vi "BallSub.vi"(6 "Ball Ref":cluster{refnum<vi>, "PaneColor":u32}[](array[cluster]), 8 "Cluster width":i32=200, 9 "Ball Nr":i32, 10 "Ball Refs":refnum<vi>[](array[refnum]), 11 "Position In":i32) -> (3 "Position out":i32)   [LabVIEW 2014]
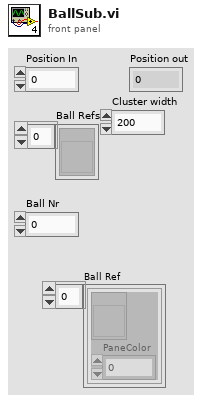
[diagram p1: front panel]
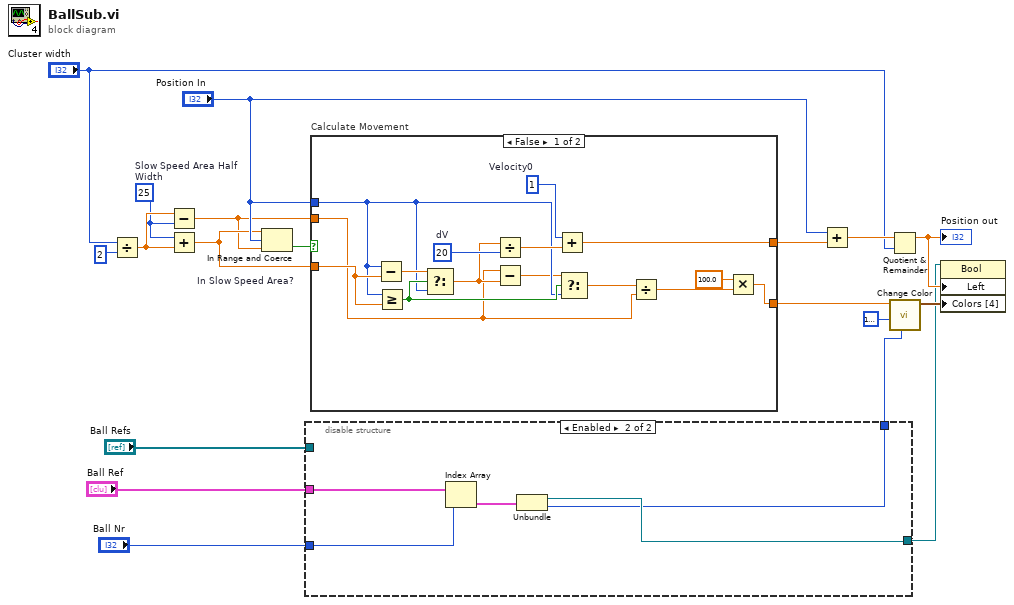
[diagram p0: block diagram]
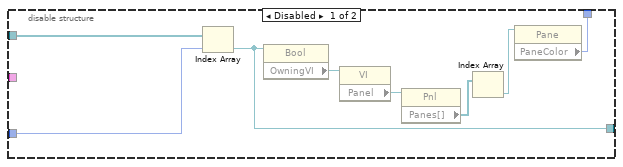
[diagram p2: hidden frame]
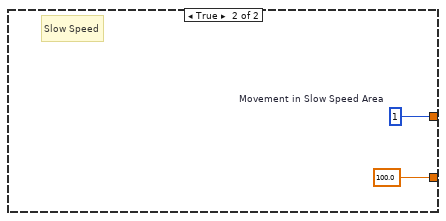
[diagram p3: hidden frame]
diagram:
  w8 = 25  # Slow Speed Area Half Width
  n1 = Divide(x="Cluster width", y=2) -> (x/y=w10:dbl)
  n2 = Subtract(x=w10, y=w8) -> (x-y=w7:dbl)
  n3 = Add(x=w8, y=w10) -> (x+y=w12:dbl)
  n4 = In Range and Coerce "In Slow Speed Area?"(upper limit=w12, x="Position In", lower limit=w7) -> (In Range?=w15:bool)  [unwired: 1 out]
  n5 = disable-structure shown="Enabled" {
    disable-tunnel: "Ball Nr" -> [w27 w31]
    disable-tunnel: "Ball Refs" -> [w26 _]
    disable-tunnel: [w21 w28] -> w3
    disable-tunnel: [w20 w29] -> w2
    disable-tunnel: "Ball Ref" -> [_ w32]
    frame Disabled {
      n6 = Index Array(array=w26, index=w27) -> (element=w20:refnum<vi>)
      n7 = property class="Bool"(reference=w20) -> ("OwningVI"=w25:refnum<vi>)  [unwired: 1 in, 2 out]
      n8 = property class="VI"(reference=w25) -> ("Panel"=w24:refnum<vi>)  [unwired: 1 in, 2 out]
      n9 = property class="Pnl"(reference=w24) -> ("Panes[]"=w23:refnum<vi>[])  [unwired: 1 in, 2 out]
      n10 = Index Array(array=w23) -> (element=w22:refnum<vi>)  [unwired: 1 in]
      n11 = property class="Pane"(reference=w22) -> ("PaneColor"=w21:u32)  [unwired: 1 in, 2 out]
    }
    frame Enabled {
      n12 = Index Array(array=w32, index=w31) -> (element=w30:cluster{refnum<vi>, "PaneColor":u32})
      n13 = Unbundle(w30) -> (w29:refnum<vi>, "PaneColor"=w28:u32)
    }
  }
  n14 = case "Calculate Movement" shown="False" w15 {
    tunnel: [w46 w49] -> w16
    tunnel: "Position In" -> [w40 _]
    tunnel: w12 -> [w44 _]
    tunnel: w7 -> [w36 _]
    tunnel: [w33 100.0] -> w4
    frame False {
      w45 = 20  # dV
      w47 = 1  # Velocity0
      n15 = Subtract(x=w40, y=w44) -> (x-y=w43:dbl)
      n16 = Greater Or Equal?(x=w40, y=w44) -> (x >= y?=w41:bool)
      n17 = Select(t=w43, s=w41, f=w40) -> (s? t:f=w39:dbl)
      n18 = Divide(x=w39, y=w45) -> (x/y=w42:dbl)
      n19 = Subtract(x=w36, y=w39) -> (x-y=w38:dbl)
      n20 = Add(x=w47, y=w42) -> (x+y=w46:dbl)
      n21 = Select(t=w38, s=w41, f=w40) -> (s? t:f=w37:dbl)
      n22 = Divide(x=w37, y=w36) -> (x/y=w35:dbl)
      n23 = Multiply(x=100.0, y=w35) -> (x*y=w33:dbl)
    }
    frame True {
      w49 = 1  # Movement in Slow Speed Area
      # "Slow Speed"
    }
  }
  n24 = Add(x="Position In", y=w16) -> (x+y=w14:dbl)
  n25 = Quotient & Remainder(x=w14, y="Cluster width") -> (x-y*floor(x/y)=w13:dbl)  [unwired: 1 out]
  "Position out" <- w13
  n26 = call "Change Color.vi"("Back Ground Color"=w3, "Current Color"=u32 16777224 ("Color"), "Color Strength (%)"=w4) -> ("output array"=w6:cluster{"Color":u32, "Color":u32}[])  [unwired: 8 out]
  n27 = property class="Bool"(reference=w2, "Left"=w13, "Colors [4]"=w6) -> ()  [unwired: 1 in, 2 out]
